vi "Update Button Images.vi"(4 "New Index":i32=-1, 6 "Old Index":i32=-1, 7 "Force Regen":bool, 8 "error in (no error)":errorcluster, 9 "Old State":T1={"Buttons Displayed"=0, "Button States"=[], "Button Size"=0, "Button Style"=enum."Classic", "Active Button"=0, "Force Regen?"=FALSE, "Tip String Ref"=refnum} caption="State", 10 "New State":T1={"Buttons Displayed"=0, "Button States"=[], "Button Size"=0, "Button Style"=enum."Classic", "Active Button"=0, "Force Regen?"=FALSE, "Tip String Ref"=refnum} caption="State", 11 "Images In":picture[](array[picture])) -> (0 "error out":errorcluster, 2 "State Out":T1={"Buttons Displayed"=0, "Button States"=[], "Button Size"=0, "Button Style"=enum."Classic", "Active Button"=0, "Force Regen?"=FALSE, "Tip String Ref"=refnum} caption="State", 3 "Images Out":picture[](array[picture]))   [LabVIEW 2012, in "Toolbar.xctl"]
doc: "Works out a new button image, either completely regenerating the image from the drawing data or if it can, just by switching between the pre-cached images for each state."
uses:
  Toolbar.xctl
  Toolbar State.ctl
  Button_Class/Button.lvclass
  Button_Class/Type Defs/Button Style.ctl
  <vilib>/Analysis/1siggen.llb/Ramp Pattern by Samples.vi
  <vilib>/Analysis/NI_AALBase.lvlib
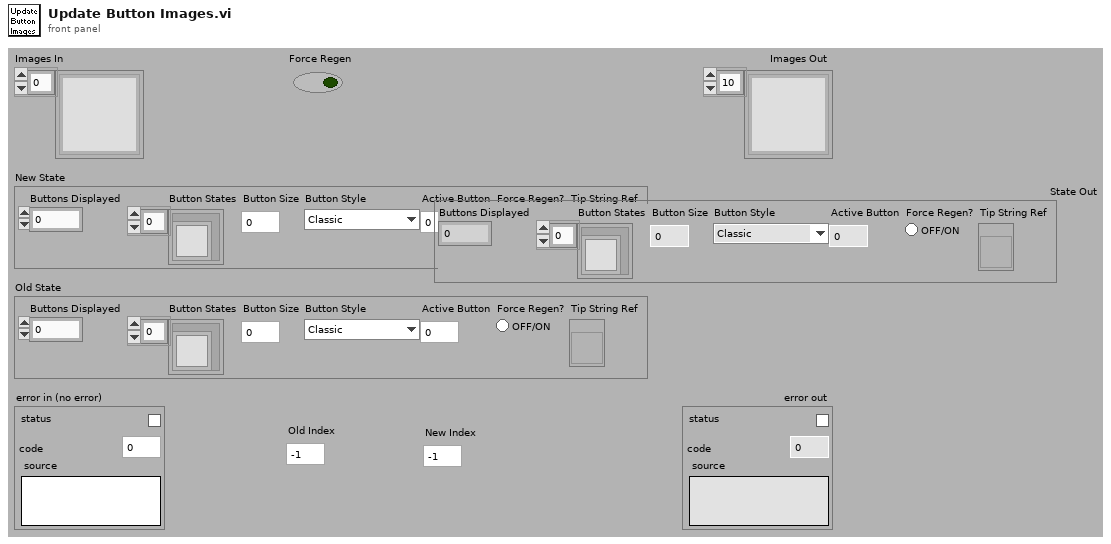
[diagram p1: front panel]
types:
  T1 = typedef "Toolbar.xctl/Toolbar State.ctl" = cluster{"Buttons Displayed":i32, "Button States":refnum<class "Button.lvclass">[], "Button Size":i32, "Button Style":T2, "Active Button":i32, "Force Regen?":bool, "Tip String Ref":refnum<vi>}
  T2 = typedef "Button.lvclass/Button Style.ctl" = enum16{"System", "Modern", "Classic", "Rounded", "Silver", "Ni Theme", "Metallic"}
  T3 = typedef "Button.lvclass/Button Status.ctl" = enum16{"Off", "Hover", "On", "Disabled"}
  T4 = typedef "Button.lvclass/Button Type.ctl" = enum16{"Transitory", "Latching"}
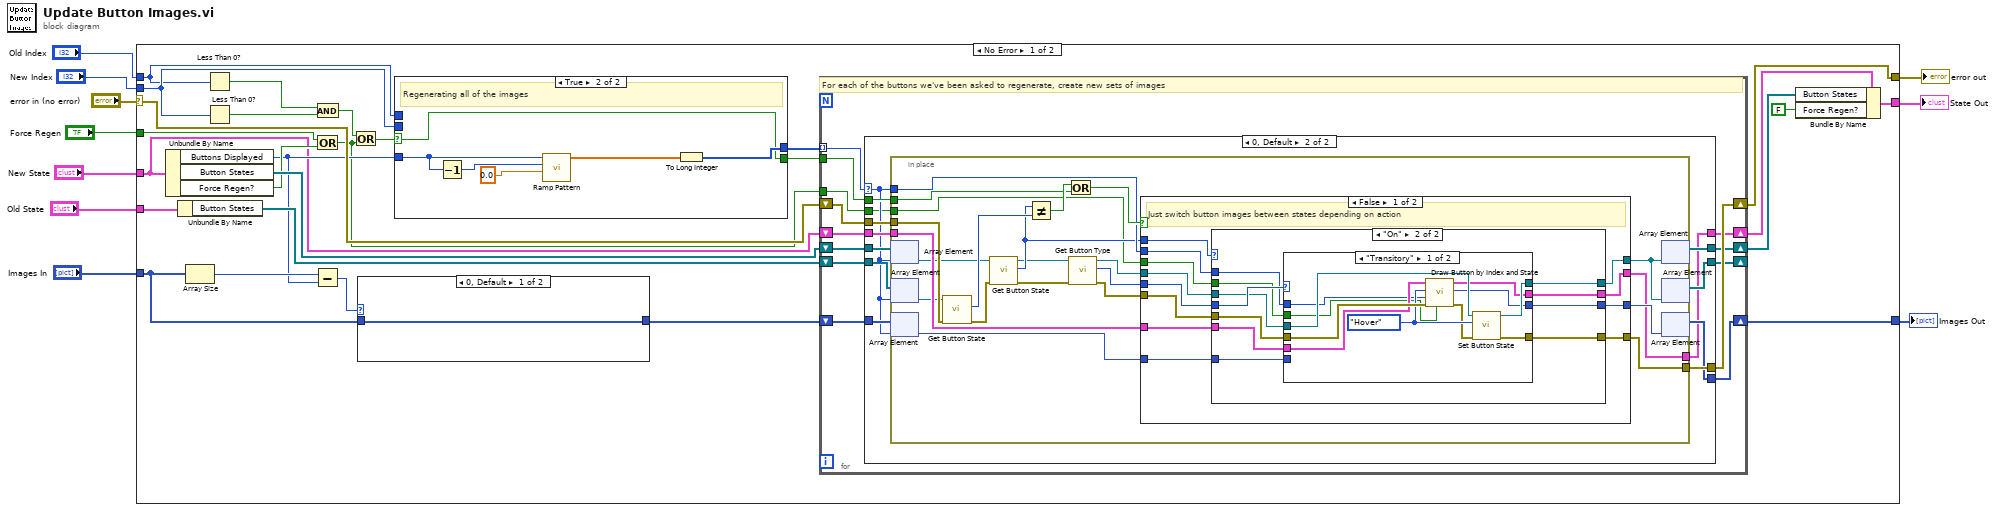
[diagram p0: block diagram]
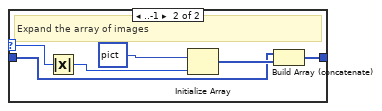
[diagram p2: hidden frame]
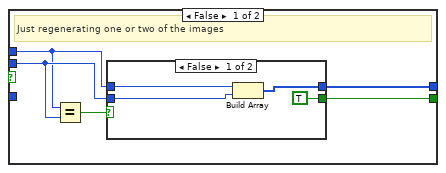
[diagram p3: hidden frame]
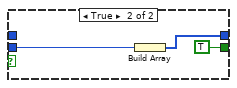
[diagram p4: hidden frame]
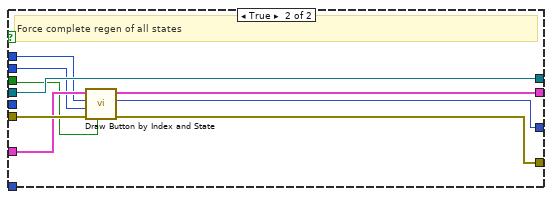
[diagram p8: hidden frame]
diagram:
  n1 = case shown="No Error" "error in (no error)" {
    selector: "error in (no error)" -> [w35 w168]
    tunnel: "New State" -> [w16 w167]
    tunnel: [w34 w168] -> w9
    tunnel: "Old State" -> [w37 _]
    tunnel: "Images In" -> [w18 _]
    tunnel: [w36 _] -> w7
    tunnel: [w33 w167] -> w6
    tunnel: "Force Regen" -> [w24 _]
    tunnel: "New Index" -> [w12 _]
    tunnel: "Old Index" -> [w11 _]
    frame No Error {
      n2 = Unbundle By Name(w16) -> ("Buttons Displayed"=w20:i32, "Button States"=w30:refnum<class "Button.lvclass">[], "Force Regen?"=w23:bool)
      n3 = Unbundle By Name(w37) -> ("Button States"=w31:refnum<class "Button.lvclass">[])
      n4 = Array Size(array=w18) -> (size(s)=w21:i32)
      n5 = Less Than 0?(x=w11) -> (x < 0?=w28:bool)
      n6 = Less Than 0?(x=w12) -> (x < 0?=w27:bool)
      n7 = Or(x=w24, y=w23) -> (x .or. y?=w13:bool)
      n8 = Subtract(x=w21, y=w20) -> (x-y=w19:i32)
      n9 = And(x=w28, y=w27) -> (x .and. y?=w26:bool)
      n10 = Or(x=w26, y=w13) -> (x .or. y?=w14:bool)
      n11 = case shown="0, Default" w19 {
        selector: w19 -> [_ w43]
        tunnel: w18 -> [w38 w40]
        tunnel: [w38 w39] -> w17
        frame 0, Default {
        }
        frame ..-1 {
          # "Expand the array of images"
          n12 = Absolute Value(x=w43) -> (abs(x)=w44:i32)
          n13 = Initialize Array(picture data[5B] ("On Picture"), w44) -> (w41:picture[])
          n14 = Build Array (concatenate)(w40, w41) -> (w39:picture[])
        }
      }
      n15 = case shown="True" w14 {
        selector: w14 -> [_ w57]
        tunnel: w20 -> [_ w61]
        tunnel: [w49 w58] -> w29
        tunnel: w11 -> [w46 _]
        tunnel: w12 -> [w47 _]
        tunnel: [w48 w57] -> w25
        frame False {
          # "Just regenerating one or two of the images"
          n16 = Equal?(x=w46, y=w47) -> (x = y?=w45:bool)
          n17 = case shown="False" w45 {
            tunnel: [w53 w55] -> w49
            tunnel: [TRUE TRUE] -> w48
            tunnel: w47 -> [w51 w56]
            tunnel: w46 -> [w50 _]
            frame False {
              n18 = Build Array(w50, w51) -> (w53:i32[])
            }
            frame True {
              n19 = Build Array(w56) -> (w55:i32[])
            }
          }
        }
        frame True {
          # "Regenerating all of the images"
          n20 = Decrement(x=w61) -> (x-1=w62:i32)
          n21 = call-poly <vilib>:"Ramp Pattern.vi"("start"=0.0, "end"=w62, "samples"=w61) -> ("Ramp Pattern"=w59:dbl[])  [unwired: 7 in, 1 out]
          n22 = To Long Integer(number=w59) -> (32bit integer=w58:i32[])
        }
      }
      n23 = for {
        shift-right: [w68] -> w36
        shift-left: w17 -> [w69]
        shift-right: [w75] -> w34
        shift-left: w35 -> [w72]
        tunnel: w25 -> [w74]
        shift-right: [w70] -> w32
        shift-left: w30 -> [w71]
        tunnel: w29 -> [w65] mode=indexing
        shift-right: [w66] -> _
        shift-left: w31 -> [w67]
        shift-right: [w64] -> w15
        shift-left: w16 -> [w73]
        tunnel: w13 -> [w63]
        # "For each of the buttons we've been asked to regenerate, create new sets of images"
        n24 = case shown="0, Default" w65 {
          selector: w65 -> [_ w83]
          tunnel: [w77 w93] -> w75
          tunnel: w74 -> [_ w92]
          tunnel: w73 -> [w76 w91]
          tunnel: w72 -> [w77 w90]
          tunnel: w71 -> [w78 w89]
          tunnel: [w78 w88] -> w70
          tunnel: w69 -> [w79 w87]
          tunnel: [w79 w86] -> w68
          tunnel: w67 -> [w80 w85]
          tunnel: [w80 w84] -> w66
          tunnel: [w76 w82] -> w64
          tunnel: w63 -> [_ w81]
          frame ..-1 {
          }
          frame 0, Default {
            n25 = in-place {
              in-place-border: [w114] -> w93
              in-place-border: w92 -> [w112]
              in-place-border: w91 -> [w111]
              in-place-border: w83 -> [w110]
              in-place-border: w90 -> [w102]
              in-place-border: [w95] -> w82
              in-place-border: w81 -> [w94]
              n26 = in-place-array #1(w89, w83) -> (w100:refnum<class "Button.lvclass">)
              n27 = in-place-array #2(w85, w83) -> (w97:refnum<class "Button.lvclass">)
              n28 = in-place-array #3(w87, w83) -> (w99:picture)
              n29 = call-dynamic "Get Button State.vi"("error in (no error)"=w102, "Button in"=w97) -> ("error out"=w108:errorcluster, "State"=w109:T3)  [unwired: 8 out]
              n30 = call-dynamic "Get Button State.vi"("error in (no error)"=w108, "Button in"=w100) -> ("error out"=w105:errorcluster, "State"=w107:T3, "Button out"=w106:refnum<class "Button.lvclass">)  [unwired: 7 out]
              n31 = Not Equal?(x=w107, y=w109) -> (x != y?=w115:bool)
              n32 = Or(x=w115, y=w112) -> (x .or. y?=w113:bool)
              n33 = call-dynamic "Get Button Type.vi"("error in (no error)"=w105, "Button in"=w106) -> ("error out"=w101:errorcluster, "Type"=w103:T4, "Button out"=w104:refnum<class "Button.lvclass">)  [unwired: 7 out]
              n34 = case shown="False" w113 {
                tunnel: [w122 w164] -> w114
                tunnel: w101 -> [w123 w165]
                tunnel: w107 -> [w127 w162]
                tunnel: w104 -> [w125 w166]
                tunnel: [w124 w166] -> w96
                tunnel: w103 -> [w126 _]
                tunnel: w111 -> [w121 w163]
                tunnel: w110 -> [w120 w161]
                tunnel: w99 -> [w118 _]
                tunnel: [w119 w160] -> w98
                tunnel: [w117 w159] -> w95
                tunnel: w94 -> [w116 w158]
                frame False {
                  # "Just switch button images between states depending on action"
                  n35 = case shown="\"On\"" w127 {
                    tunnel: w125 -> [w131 w140]
                    tunnel: w126 -> [_ w142]
                    tunnel: [w131 w141] -> w124
                    tunnel: w123 -> [w130 w139]
                    tunnel: [w130 w138] -> w122
                    tunnel: w121 -> [w128 w137]
                    tunnel: w120 -> [_ w136]
                    tunnel: [w129 w135] -> w119
                    tunnel: w118 -> [w129 w134]
                    tunnel: [w128 w133] -> w117
                    tunnel: w116 -> [_ w132]
                    frame "Off", Default {
                    }
                    frame "On" {
                      n36 = case shown="\"Transitory\"" w142 {
                        tunnel: [w149 w157] -> w141
                        tunnel: w140 -> [w150 w157]
                        tunnel: w139 -> [w153 w156]
                        tunnel: [w147 w156] -> w138
                        tunnel: w137 -> [w152 w154]
                        tunnel: w136 -> [w146 _]
                        tunnel: [w145 w155] -> w135
                        tunnel: w134 -> [_ w155]
                        tunnel: [w144 w154] -> w133
                        tunnel: w132 -> [w143 _]
                        frame "Transitory" {
                          w151 = enum16{"Off", "Hover", "On", "Disabled"}."Hover" ("State")
                          n37 = call "Draw Button by Index and State.vi"("Force redraw ?"=w143, "error in (no error)"=w153, "index"=w146, "Button State"=w151, "State"=w152) -> ("error out"=w148:errorcluster, "Picture Out"=w145:picture, "State out"=w144:T1)  [unwired: 3 in, 1 out]
                          n38 = call-dynamic "Set Button State.vi"("error in (no error)"=w148, "State"=w151, "Button in"=w150) -> ("error out"=w147:errorcluster, "Button out"=w149:refnum<class "Button.lvclass">)  [unwired: 1 in, 6 out]
                        }
                        frame "Latching", Default {
                        }
                      }
                    }
                  }
                }
                frame True {
                  # "Force complete regen of all states"
                  n39 = call "Draw Button by Index and State.vi"("Force redraw ?"=w158, "error in (no error)"=w165, "index"=w161, "Button State"=w162, "State"=w163) -> ("error out"=w164:errorcluster, "Picture Out"=w160:picture, "State out"=w159:T1)  [unwired: 3 in, 1 out]
                }
              }
              n40 = in-place-array #1(w96) -> (w88:refnum<class "Button.lvclass">[])  [unwired: 1 out]
              n41 = in-place-array #2(w96) -> (w84:refnum<class "Button.lvclass">[])  [unwired: 1 out]
              n42 = in-place-array #3(w98) -> (w86:picture[])  [unwired: 1 out]
            }
          }
        }
      }
      n43 = Bundle By Name(cluster=w15, "Button States"=w32, "Force Regen?"=FALSE) -> (w33:T1)
    }
    frame Error {
    }
  }
  "Images Out" <- w7
  "error out" <- w9
  "State Out" <- w6
